vi "LVObject to JSON - Malicious Serialization Binder - Escapes Malicious JSON.vi"() -> ()   [LabVIEW 2017, in "Generic Object Serializer Tests.lvlib" / "Serialization Binder.lvlib"]
uses:
  Serialization Binder.lvlib
  Generic Object Serializer/Generic Object Serializer.lvclass
  Malicious Serialization Binder/Malicious Serialization Binder.lvclass
  C:/Users/de200256/Code/logmanoriginal/jsontext-object-serialization/Serialization Binder/Serialization Binder.lvclass
  Generic Object Serializer/Type Name Handling.ctl
  Generic Object Serializer/Generic Object Serializer.lvclass/Generic Object Serializer.ctl
  Generic Object Serializer/Write Serialization Binder.vi
  Generic Object Serializer/Write Type Name Handling.vi
  <vilib>/addons/_JKI Toolkits/Caraya/classes/Test/Test.lvclass
  <vilib>/addons/_JKI Toolkits/Caraya/classes/Assert/Assert.lvclass
panel:
  out "error out":errorcluster
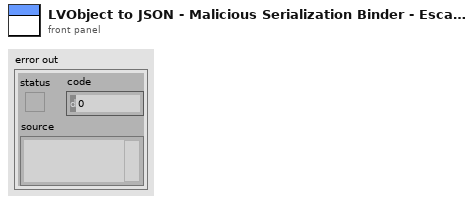
[diagram p1: front panel]
types:
  T1 = typedef "Generic Object Serializer.lvclass/Type Name Handling.ctl" = enum16{"None", "Inline"}
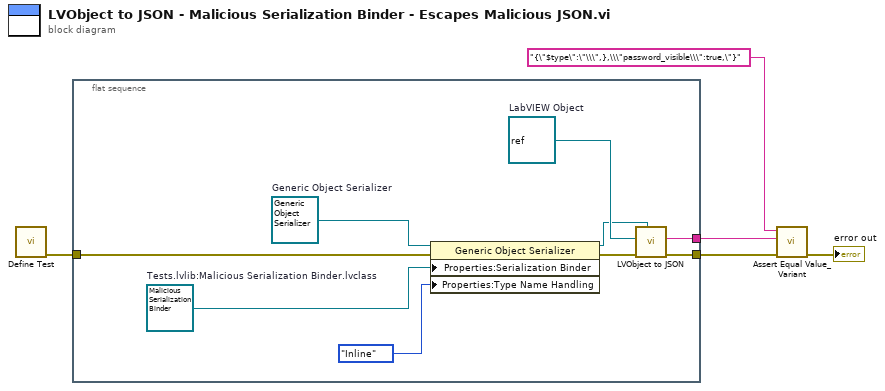
[diagram p0: block diagram]
diagram:
  n1 = call <vilib>:"Define Test.vi"() -> ("error out"=w5:errorcluster)  [unwired: 11 in]
  n2 = flat-sequence {
    tunnel: [w7] -> w4
    tunnel: w5 -> [w13]
    tunnel: [w6] -> w2
    frame #0 {
      w11 = refnum<class> refnum  # LabVIEW Object
      w12 = refnum<class "Malicious Serialization Binder.lvclass"> refnum  # Tests.lvlib:Malicious Serialization Binder.lvclass
      w14 = refnum<class "Generic Object Serializer.lvclass"> refnum  # Generic Object Serializer
      n3 = property class="Generic Object Serializer"(reference=w14, error in=w13, "Properties:Serialization Binder"=w12, "Properties:Type Name Handling"=Type_Name_Handling."Inline" ("Type Name Handling")) -> (reference out=w10:refnum<class "Generic Object Serializer.lvclass">, error out=w8:errorcluster)
      n4 = call-dynamic "LVObject to JSON.vi"("LVClass Serializer"=w10, "error in (no error)"=w8, "Object"=w11) -> ("error out"=w7:errorcluster, "<JSON>Object"=w6:string)  [unwired: 7 in]
    }
  }
  n5 = call <vilib>:"Assert Equal Value_Variant.vi"("error in (no error)"=w4, "Y"=w2, "X"="{\"$type\":\"\\\",},\\\"password_visible\\\":true,\"}" ("<JSON>Object")) -> ("error out"=→"error out":errorcluster)  [unwired: 8 in]
